vi "round to binary 10s.vi"(11 "Numeric":u32 format="%b") -> (3 "Numeric 2":u32 format="%b")   [LabVIEW 2016]
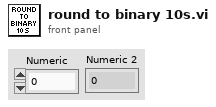
[diagram p1: front panel]
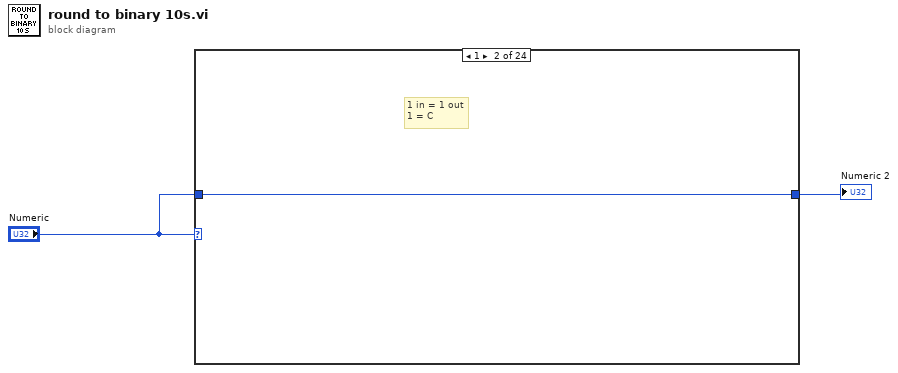
[diagram p0: block diagram]
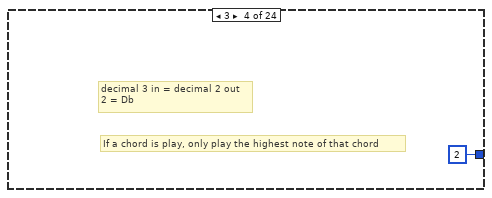
[diagram p4: hidden frame]
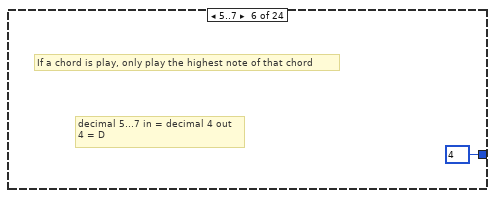
[diagram p6: hidden frame]
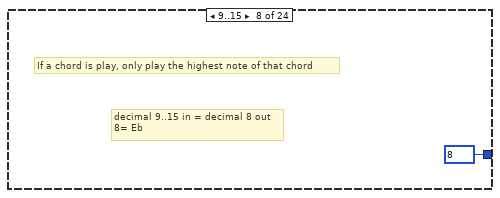
[diagram p8: hidden frame]
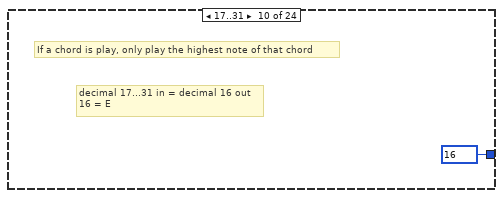
[diagram p10: hidden frame]
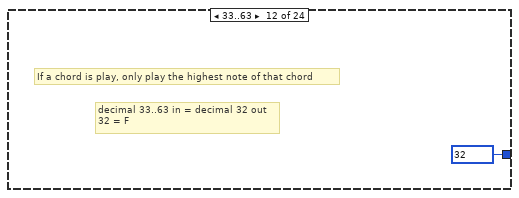
[diagram p12: hidden frame]
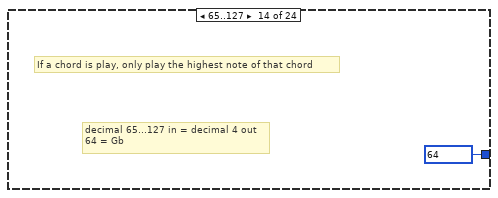
[diagram p14: hidden frame]
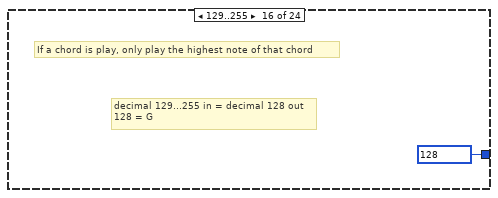
[diagram p16: hidden frame]
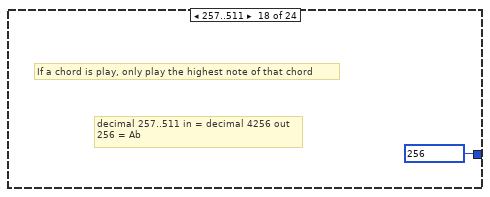
[diagram p18: hidden frame]
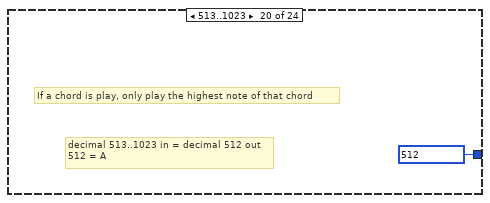
[diagram p20: hidden frame]
diagram:
  n1 = case shown="1" "Numeric" {
    tunnel: [w3 w4 w5 u32 2 ("Numeric") w7 u32 4 ("Numeric") w9 u32 8 ("Numeric") w11 u32 16 ("Numeric") w13 u32 32 ("Numeric") w15 u32 64 ("Numeric") w17 u32 128 ("Numeric") w19 u32 256 ("Numeric") w21 u32 512 ("Numeric") w23 u32 1024 ("Numeric") w25 u32 2048 ("Numeric")] -> w2
    tunnel: "Numeric" -> [w3 w4 w5 _ w7 _ w9 _ w11 _ w13 _ w15 _ w17 _ w19 _ w21 _ w23 _ w25 _]
    frame 0, Default {
      # "0 in = 0 out\n0 means no note played"
    }
    frame 1 {
      # "1 in = 1 out\n1 = C"
    }
    frame 2 {
      # "decimal 2 in = decimal 2 out\n2 = Db"
    }
    frame 3 {
      # "If a chord is play, only play the highest note of that chord"
      # "decimal 3 in = decimal 2 out\n2 = Db"
    }
    frame 4 {
      # "decimal 4 in = decimal 4 out\n4 = D"
    }
    frame 5..7 {
      # "decimal 5...7 in = decimal 4 out\n4 = D"
      # "If a chord is play, only play the highest note of that chord"
    }
    frame 8 {
      # "decimal 8 in = decimal 8 out\n8 = Eb"
    }
    frame 9..15 {
      # "decimal 9..15 in = decimal 8 out\n8= Eb"
      # "If a chord is play, only play the highest note of that chord"
    }
    frame 16 {
      # "decimal 16 in = decimal 16 out\n16 = E"
    }
    frame 17..31 {
      # "decimal 17...31 in = decimal 16 out\n16 = E"
      # "If a chord is play, only play the highest note of that chord"
    }
    frame 32 {
      # "decimal 32 in = decimal 32 out\n32 = F"
    }
    frame 33..63 {
      # "If a chord is play, only play the highest note of that chord"
      # "decimal 33..63 in = decimal 32 out\n32 = F"
    }
    frame 64 {
      # "decimal 64 in = decimal 64 out\n64 = Gb"
    }
    frame 65..127 {
      # "decimal 65...127 in = decimal 4 out\n64 = Gb"
      # "If a chord is play, only play the highest note of that chord"
    }
    frame 128 {
      # "decimal 128 in = decimal 128 out\n128 = G"
    }
    frame 129..255 {
      # "decimal 129...255 in = decimal 128 out\n128 = G"
      # "If a chord is play, only play the highest note of that chord"
    }
    frame 256 {
      # "decimal 256 in = decimal 256 out\n256 = Ab"
    }
    frame 257..511 {
      # "decimal 257..511 in = decimal 4256 out\n256 = Ab"
      # "If a chord is play, only play the highest note of that chord"
    }
    frame 512 {
      # "decimal 512 in = decimal 512 out\n512 = A"
    }
    frame 513..1023 {
      # "decimal 513..1023 in = decimal 512 out\n512 = A"
      # "If a chord is play, only play the highest note of that chord"
    }
    frame 1024 {
      # "decimal 1024 in = decimal 1024 out\n1024 = Bb"
    }
    frame 1025..2047 {
      # "decimal 1025..2047 in = decimal 1024 out\n1024 = Bb"
      # "If a chord is play, only play the highest note of that chord"
    }
    frame 2048 {
      # "decimal 2048 in = decimal 2048 out\n2048 = B"
    }
    frame 2049..16383 {
      # "decimal 2049..end in = decimal 2048 out\n2048 = B"
      # "If a chord is play, only play the highest note of that chord"
    }
  }
  "Numeric 2" <- w2
